vi "CTE_Analysis_Suite_InputMaker_FormatStringS.vi"(8 "VALUE":dbl, 11 "NAME":string) -> (3 "Output":string)   [LabVIEW 2012]
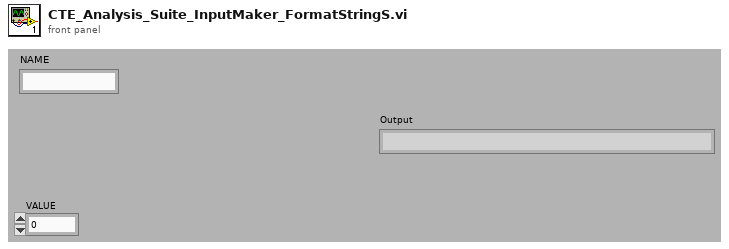
[diagram p1: front panel]
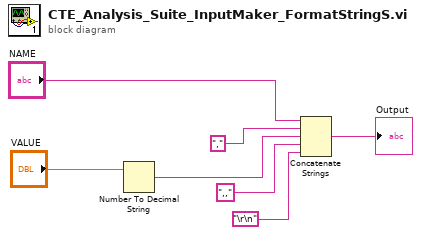
[diagram p0: block diagram]
diagram:
  n1 = Number To Decimal String(number="VALUE") -> (decimal integer string=w6:string)  [unwired: 1 in]
  n2 = Concatenate Strings("NAME", ",", w6, ",,", "\r\n") -> (→"Output":string)
